vi "DCPower_ParameterCreation.vi"(2 "error in":errorcluster caption="error out", 3 "Precision":string, 4 "DCPowerInformationByInstrument":T1) -> (0 "error out":errorcluster, 1 "DCPowerInfoArray":string[][](array[string]))   [LabVIEW 2019]
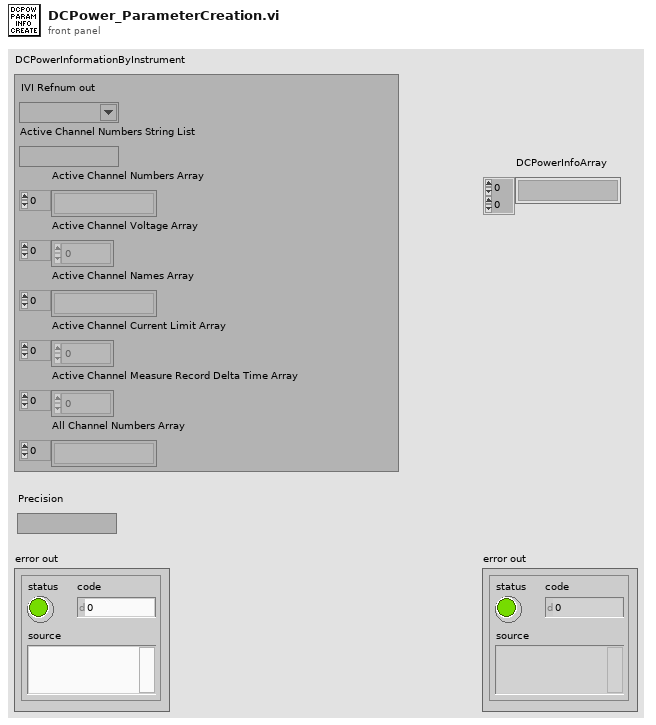
[diagram p1: front panel]
types:
  T1 = cluster{"IVI Refnum out":refnum<k15>, "Active Channel Numbers String List":string, "Active Channel Numbers Array":string[], "Active Channel Voltage Array":dbl[], "Active Channel Names Array":string[], "Active Channel Current Limit Array":dbl[], "Active Channel Measure Record Delta Time Array":dbl[], "All Channel Numbers Array":string[]}
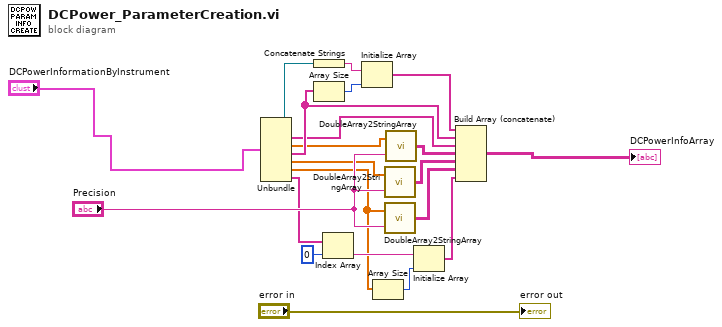
[diagram p0: block diagram]
diagram:
  n1 = Unbundle("DCPowerInformationByInstrument") -> ("IVI Refnum out"=w19:refnum<k15>, "Active Channel Numbers Array"=w10:string[], "Active Channel Voltage Array"=w14:dbl[], "Active Channel Names Array"=w17:string[], "Active Channel Current Limit Array"=w15:dbl[], "Active Channel Measure Record Delta Time Array"=w3:dbl[], "All Channel Numbers Array"=w6:string[])  [unwired: 1 out]
  n2 = Concatenate Strings(w19) -> (w20:string)
  n3 = Array Size(array=w17) -> (size(s)=w18:i32)
  n4 = Index Array(array=w6, index=0) -> (element=w4:string)
  n5 = Initialize Array(w20, w18) -> (w21:string[])
  n6 = Array Size(array=w3) -> (size(s)=w2:i32)
  n7 = call "DoubleArray2StringArray.vi"("Precision"="Precision", "Double Array Input"=w15) -> ("STring Array Output"=w12:string[][])
  n8 = call "DoubleArray2StringArray.vi"("Precision"="Precision", "Double Array Input"=w3) -> ("STring Array Output"=w13:string[][])
  n9 = call "DoubleArray2StringArray.vi"("Precision"="Precision", "Double Array Input"=w14) -> ("STring Array Output"=w11:string[][])
  n10 = Initialize Array(w4, w2) -> (w1:string[])
  n11 = Build Array (concatenate)(w21, w17, w10, w11, w12, w13, w1) -> (→"DCPowerInfoArray":string[][])
  "error out" <- "error in"
